vi "Data Logging - DAQ 9172.vi"() -> ()   [LabVIEW 2016]
uses:
  <vilib>/express/express shared/transition.llb/Dynamic To Waveform Array.vi
  <vilib>/express/express arith-compare/Formula/Block/exnFormulaBlock how many pts in the wave.vi
  <vilib>/express/express shared/ex_Modify Signal Name.vi
  <vilib>/express/express shared/transition.llb/Waveform Array To Dynamic.vi
  <vilib>/express/express arith-compare/Formula/XNode/ExpressFormulaBlockNode.xnode
panel:
  out "Raw History":dynamicdata(graph)
  out "Relative Saturation (%)":dynamicdata(graph)
  out "RS Vaisala":dbl
  out "PPM H2O2":dynamicdata(graph)
  out "PPM ATI":dbl
  out "PPM Vaisala":dbl
  out "Raw Data":dynamicdata(graph)
  in  "stop (F)":bool
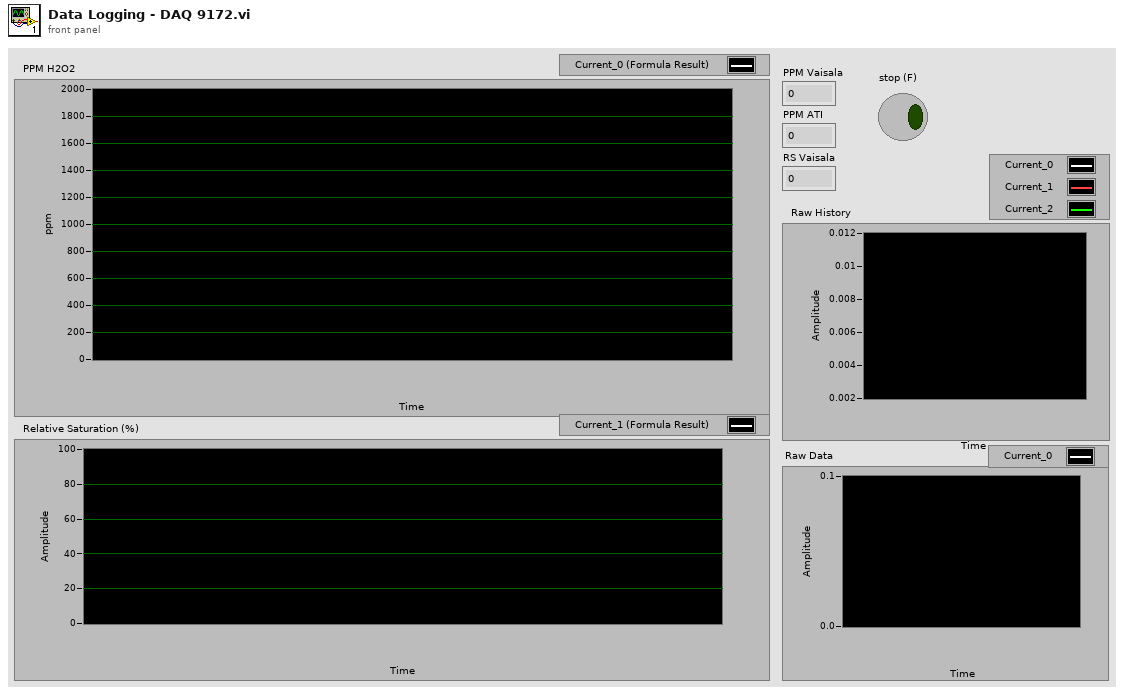
[diagram p1: front panel]
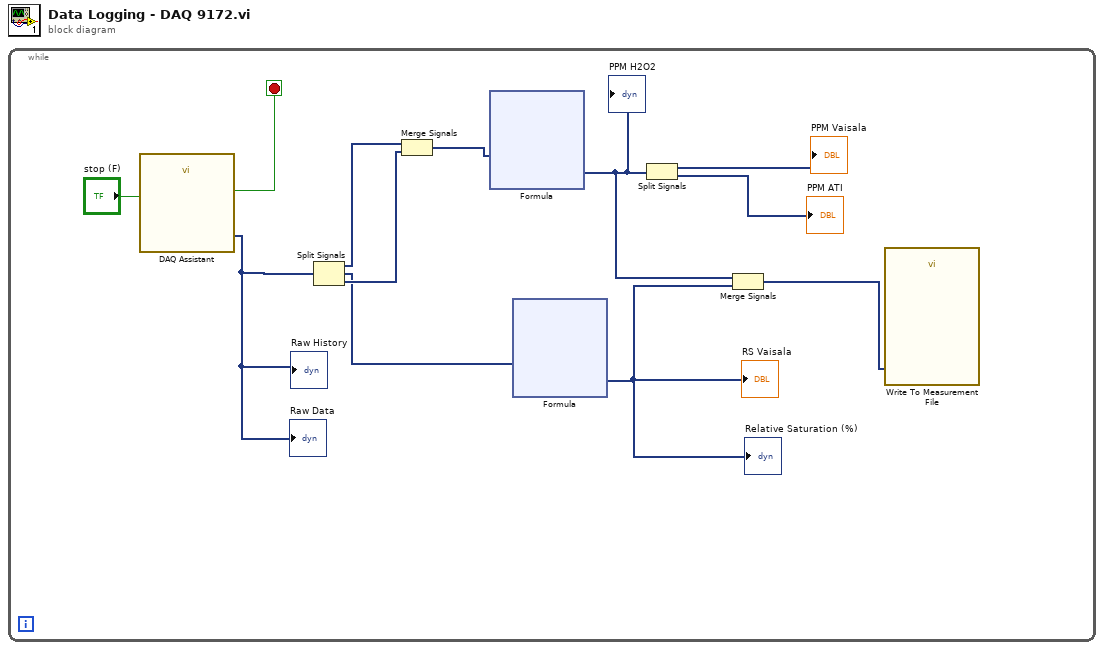
[diagram p0: block diagram]
diagram:
  n1 = while {
    stop <- w11 stop-if-true
    n2 = call "DAQ Assistant"("stop (F)"="stop (F)") -> ("data"=w1:dynamicdata, "stopped"=w11:bool)  [unwired: 15 in, 2 out]
    "Raw Data" <- w1
    "Raw History" <- w1
    n3 = Split Signals(w1) -> (w10:dynamicdata, w7:dynamicdata, w9:dynamicdata)  [unwired: 3 in]
    n4 = Merge Signals(w10, w9) -> (w8:dynamicdata)
    n5 = xnode "Formula"("AI1"=w8) -> ("Result"=w4:dynamicdata)  [unwired: 1 in, 1 out]
    "PPM H2O2" <- w4
    n6 = xnode "Formula"("AI2"=w7) -> ("Result"=w3:dynamicdata)  [unwired: 1 in, 1 out]
    "RS Vaisala" <- w3
    "Relative Saturation (%)" <- w3
    n7 = Split Signals(w4) -> (→"PPM Vaisala":dynamicdata, →"PPM ATI":dynamicdata)  [unwired: 2 in]
    n8 = Merge Signals(w4, w3) -> (w2:dynamicdata)
    n9 = call "Write To Measurement File"("Signals"=w2) -> ()  [unwired: 16 in, 3 out]
  }
